vi "Calibration_Capture.vi"(8 "Detect Movement":bool, 9 "Crop?":bool, 11 "value":T1={"Pinch-valve"="Test Sample", "XLP 6000 Pump"="MRJ", "Camera1"="", "Camera2"="", "Img_Capt"=FALSE, "Actuator"=FALSE, "Pump"=FALSE, "Cam 1"=FALSE, "Cam 2"=FALSE, "Empty_Refill"=FALSE, "Crop"=FALSE, "Light intensity"=0, "Exposure Time"=0.0, "Sample Name"="", "Operator"="JFR", "Calibration 1"=path "C:/Users/au540322/Desktop/IHS_Project/images/Debris/Debris_0/Debris_0_2019_06_01-23-32-49-686.PNG", "Calibration 2"=path "C:/Users/au540322/Desktop/IHS_Project/images/Debris/Debris_0/Debris_0_2019_06_01-23-32-49-686.PNG", "Framerate"=15, "Timeout Sample"=1, "Collection date"="", "Sample size threshold"=500, "Empty start"=500, "Command"="", "Station"="", "Species Name"="", "Other Notes"="", "Aperture"=enum."Item 3", "Image Process Queue Size"=100, "Image Save Queue Size"=0, "Overload threshold"=0, "Max Framerate"=0, "Rectangle 1"={"Left"=0, "Top"=0, "Right"=0, "Bottom"=0, "Rotation"=0.0}, "Rectangle 2"={"Left"=0, "Top"=100, "Right"=100, "Bottom"=0, "Rotation"=0.0}, "Detection Region %"=200.0, "Detect 1"=path "C:/Users/au540322/Desktop/IHS_Project/images/Debris/Debris_0/Debris_0_2019_06_01-23-32-49-686.PNG", "Detect 2"=path "C:/Users/au540322/Desktop/IHS_Project/images/Debris/Debris_0/Debris_0_2019_06_01-23-32-49-686.PNG", "Max large object threshold"=500, "Open(T)/Close(F)"=FALSE, "Img_Capt Begin"=FALSE, "Dispense Speed"=0, "Flush Size"=0, "Location"="", "Latitude"="", "Longitude"="", "Determiner"="", "Sex"="", "Camera1_Img"=refnum, "Camera2_Img"=refnum, "Img1_Orig_Disp"=refnum, "Img2_Orig_Disp"=refnum, "Img1_Orig_RGB"=refnum, "Img2_Orig_RGB"=refnum, "Blue_Plane_Extract"=refnum, "Subtracted_Plane"=refnum, "Img1_Binary"=refnum, "Img2_Binary"=refnum, "Crop_Mask"=refnum, "Img1_Save"=refnum, "Img2_Save"=refnum, "Img1_Cali_Full"=refnum, "Img2_Cali_Full"=refnum, "Img1_Cali_Detect"=refnum, "Img2_Cali_Detect"=refnum, "Cam 1 queue"=refnum, "Cam 2 queue"=refnum, "Cam 1 - save queue"=refnum, "Cam 2 - save queue"=refnum, "Overlay_Ring"=0, "SystemVersion"=0, "System Serial"="", "Legacy Cam Attributes"=FALSE, "Camera Orientation 1"="", "Camera Orientation 2"="", "Pixel to mm 1"=0.0, "Pixel to mm 2"=0.0, "CAM1 Model"=enum."a2A5328-15ucBAS", "CAM2 Model"=enum."a2A5328-15ucBAS", "Flush Insect"=FALSE, "Pump Size"=TRUE, "Barcode"="", "Phase3"=FALSE, "Mega F3"="", "Container nr."=0.0, "Flush Error"=TRUE, "Start System"=FALSE, "Size Interval"=0.0, "Mun. of containers"=0.0, "Sorting sys."=FALSE, "Initial size"=0.0} {"SystemVersion" items=["Standard", "XL"]; "Overlay_Ring" items=["Session Data", "Extended Setup", "Buffer", "Camera", "Dispenser", "Stats", "Connections"]; "Flush Size" min=1; "Dispense Speed" min=1; "Rectangle 2"."Rotation" format="%.2f"; "Rectangle 2"."Left" scale=0.0..1024.0; "Rectangle 2"."Right" scale=0.0..1024.0; "Rectangle 1"."Rotation" format="%.2f"; "Rectangle 1"."Left" scale=0.0..1024.0; "Rectangle 1"."Right" scale=0.0..1024.0; "Max Framerate" min=1; "Overload threshold" min=1; "Image Save Queue Size" min=1; "Image Process Queue Size" min=1; "Empty start" min=1; "Sample size threshold" min=1; "Framerate" min=1; "Light intensity" scale=0.0..100.0}) -> (0 "Image2":T4, 1 "Image1":T4, 3 "input cluster 2":T1={"Pinch-valve"="", "XLP 6000 Pump"="", "Camera1"="", "Camera2"="", "Img_Capt"=FALSE, "Actuator"=FALSE, "Pump"=FALSE, "Cam 1"=FALSE, "Cam 2"=FALSE, "Empty_Refill"=FALSE, "Crop"=FALSE, "Light intensity"=100, "Exposure Time"=1000.0, "Sample Name"="Test Sample", "Operator"="JFR", "Calibration 1"=path "C:/Users/au540322/Desktop/IHS_Project/images/Debris/Debris_0/Debris_0_2019_06_01-23-32-49-686.PNG", "Calibration 2"=path "C:/Users/au540322/Desktop/IHS_Project/images/Debris/Debris_0/Debris_0_2019_06_01-23-32-49-686.PNG", "Framerate"=15, "Timeout Sample"=200, "Collection date"="", "Sample size threshold"=500, "Empty start"=1, "Command"="", "Station"="", "Species Name"="", "Other Notes"="", "Aperture"=enum."Item 0", "Image Process Queue Size"=500, "Image Save Queue Size"=500, "Overload threshold"=500, "Max Framerate"=100, "Rectangle 1"={"Left"=0, "Top"=0, "Right"=0, "Bottom"=0, "Rotation"=0.0}, "Rectangle 2"={"Left"=0, "Top"=0, "Right"=0, "Bottom"=0, "Rotation"=0.0}, "Detection Region %"=0.0, "Detect 1"=path "C:/Users/au540322/Desktop/IHS_Project/images/Debris/Debris_0/Debris_0_2019_06_01-23-32-49-686.PNG", "Detect 2"=path "C:/Users/au540322/Desktop/IHS_Project/images/Debris/Debris_0/Debris_0_2019_06_01-23-32-49-686.PNG", "Max large object threshold"=0, "Open(T)/Close(F)"=FALSE, "Img_Capt Begin"=FALSE, "Dispense Speed"=100, "Flush Size"=100, "Location"="Station", "Latitude"="Station", "Longitude"="Station", "Determiner"="Station", "Sex"="Station", "Camera1_Img"=refnum, "Camera2_Img"=refnum, "Img1_Orig_Disp"=refnum, "Img2_Orig_Disp"=refnum, "Img1_Orig_RGB"=refnum, "Img2_Orig_RGB"=refnum, "Blue_Plane_Extract"=refnum, "Subtracted_Plane"=refnum, "Img1_Binary"=refnum, "Img2_Binary"=refnum, "Crop_Mask"=refnum, "Img1_Save"=refnum, "Img2_Save"=refnum, "Img1_Cali_Full"=refnum, "Img2_Cali_Full"=refnum, "Img1_Cali_Detect"=refnum, "Img2_Cali_Detect"=refnum, "Cam 1 queue"=refnum, "Cam 2 queue"=refnum, "Cam 1 - save queue"=refnum, "Cam 2 - save queue"=refnum, "Overlay_Ring"=0, "SystemVersion"=0, "System Serial"="", "Legacy Cam Attributes"=FALSE, "Camera Orientation 1"="", "Camera Orientation 2"="", "Pixel to mm 1"=0.0, "Pixel to mm 2"=0.0, "CAM1 Model"=enum."a2A5328-15ucBAS", "CAM2 Model"=enum."a2A5328-15ucBAS", "Flush Insect"=FALSE, "Pump Size"=TRUE, "Barcode"="", "Phase3"=FALSE, "Mega F3"="", "Container nr."=0.0, "Flush Error"=FALSE, "Start System"=FALSE, "Size Interval"=0.0, "Mun. of containers"=0.0, "Sorting sys."=FALSE, "Initial size"=0.0} {"SystemVersion" items=["Standard", "XL"]; "Overlay_Ring" items=["Session Data", "Extended Setup", "Buffer", "Camera", "Dispenser", "Stats", "Connections"]; "Flush Size" min=1; "Dispense Speed" min=1; "Rectangle 2"."Rotation" format="%.2f"; "Rectangle 2"."Left" scale=0.0..1024.0; "Rectangle 2"."Right" scale=0.0..1024.0; "Rectangle 1"."Rotation" format="%.2f"; "Rectangle 1"."Left" scale=0.0..1024.0; "Rectangle 1"."Right" scale=0.0..1024.0; "Max Framerate" min=1; "Overload threshold" min=1; "Image Save Queue Size" min=1; "Image Process Queue Size" min=1; "Empty start" min=1; "Sample size threshold" min=1; "Framerate" min=1; "Light intensity" scale=0.0..100.0}, 4 "error out":errorcluster)   [LabVIEW 2024]
doc: "Takes calibration images with original camera aspect ratio."
uses:
  <vilib>/vision/Image Controls.llb/IMAQ Image.ctl
  controls/Data.ctl
  <vilib>/userDefined/High Color/IMAQdx.ctl
  <vilib>/vision/driver/IMAQdx.llb/IMAQdx Acquisition Mode.ctl
  <vilib>/vision/driver/NI_Vision_Acquisition_Software.lvlib
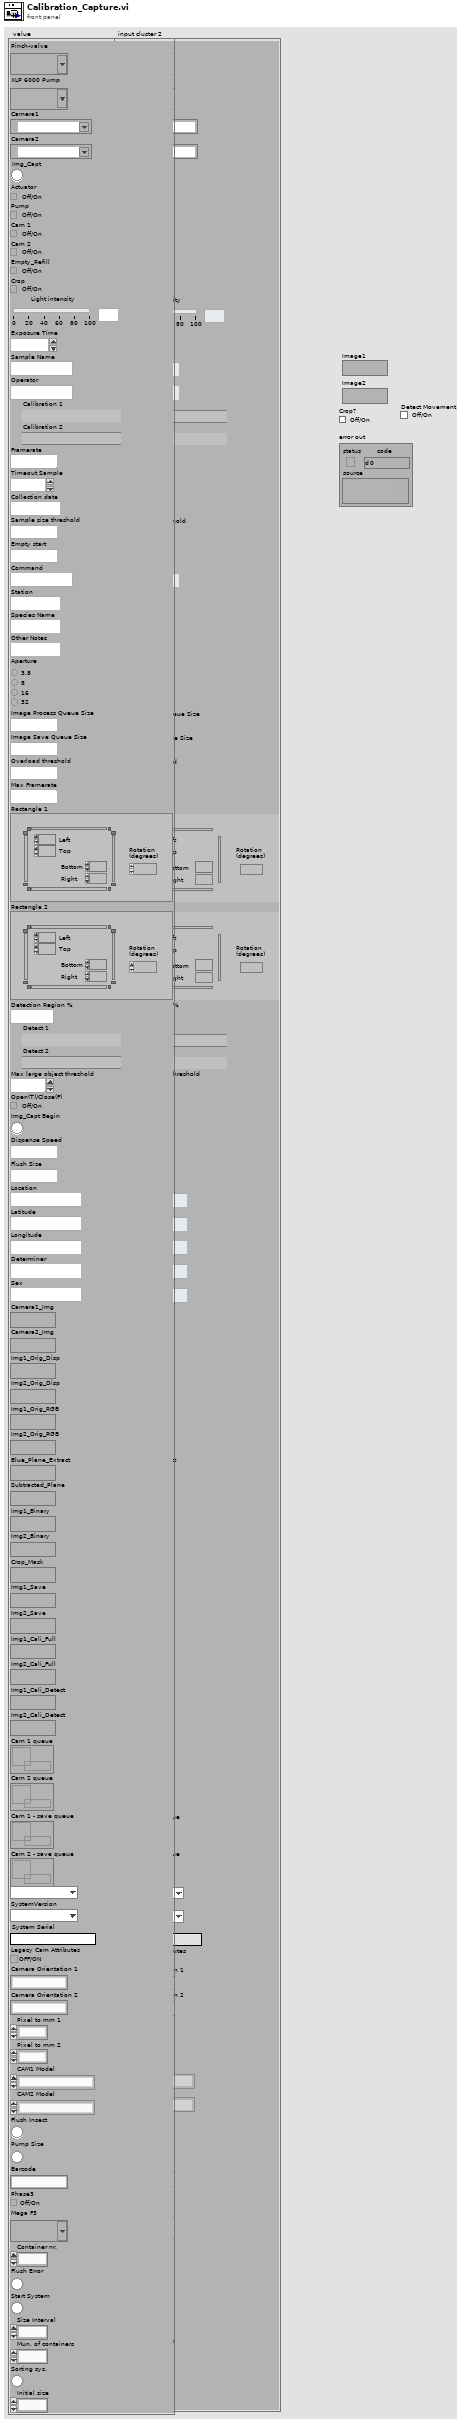
[diagram p1: front panel]
types:
  T1 = typedef "Data.ctl" = cluster{"Pinch-valve":refnum<visa-resource-name>, "XLP 6000 Pump":refnum<visa-resource-name>, "Camera1":T2, "Camera2":T2, "Img_Capt":bool, "Actuator":bool, "Pump":bool, "Cam 1":bool, "Cam 2":bool, "Empty_Refill":bool, "Crop":bool, "Light intensity":i32, "Exposure Time":dbl, "Sample Name":string, "Operator":string, "Calibration 1":path, "Calibration 2":path, "Framerate":i32, "Timeout Sample":i32, "Collection date":string, "Sample size threshold":i32, "Empty start":u32, "Command":string, "Station":string, "Species Name":string, "Other Notes":string, "Aperture":enum32{"Item 0", "Item 1", "Item 2", "Item 3"}, "Image Process Queue Size":i32, "Image Save Queue Size":i32, "Overload threshold":i32, "Max Framerate":i32, "Rectangle 1":T3, "Rectangle 2":T3, "Detection Region %":dbl, "Detect 1":path, "Detect 2":path, "Max large object threshold":i32, "Open(T)/Close(F)":bool, "Img_Capt Begin":bool, "Dispense Speed":i32, "Flush Size":i32, "Location":string, "Latitude":string, "Longitude":string, "Determiner":string, "Sex":string, "Camera1_Img":T4, "Camera2_Img":T4, "Img1_Orig_Disp":T4, "Img2_Orig_Disp":T4, "Img1_Orig_RGB":T4, "Img2_Orig_RGB":T4, "Blue_Plane_Extract":T4, "Subtracted_Plane":T4, "Img1_Binary":T4, "Img2_Binary":T4, "Crop_Mask":T4, "Img1_Save":T4, "Img2_Save":T4, "Img1_Cali_Full":T4, "Img2_Cali_Full":T4, "Img1_Cali_Detect":T4, "Img2_Cali_Detect":T4, "Cam 1 queue":refnum<queue>, "Cam 2 queue":refnum<queue>, "Cam 1 - save queue":refnum<queue>, "Cam 2 - save queue":refnum<queue>, "Overlay_Ring":u16, "SystemVersion":u16, "System Serial":string, "Legacy Cam Attributes":bool, "Camera Orientation 1":string, "Camera Orientation 2":string, "Pixel to mm 1":dbl, "Pixel to mm 2":dbl, "CAM1 Model":enum16{"a2A5328-15ucBAS", "acA1920-155uc"}, "CAM2 Model":enum16{"a2A5328-15ucBAS", "acA1920-155uc"}, "Flush Insect":bool, "Pump Size":bool, "Barcode":string, "Phase3":bool, "Mega F3":refnum<visa-resource-name>, "Container nr.":dbl, "Flush Error":bool, "Start System":bool, "Size Interval":dbl, "Mun. of containers":dbl, "Sorting sys.":bool, "Initial size":dbl}
  T2 = typedef "IMAQdx.ctl" = refnum<k21>
  T3 = typedef "IMAQ Rectangle" = cluster{"Left":i32, "Top":i32, "Right":i32, "Bottom":i32, "Rotation":dbl}
  T4 = typedef "IMAQ Image.ctl" = refnum<image>
  T5 = typedef "NI_Vision_Acquisition_Software.lvlib/IMAQdx Acquisition Mode.ctl" = enum32{"One Shot", "Continuous"}
  T6 = typedef "Image Type" = u32
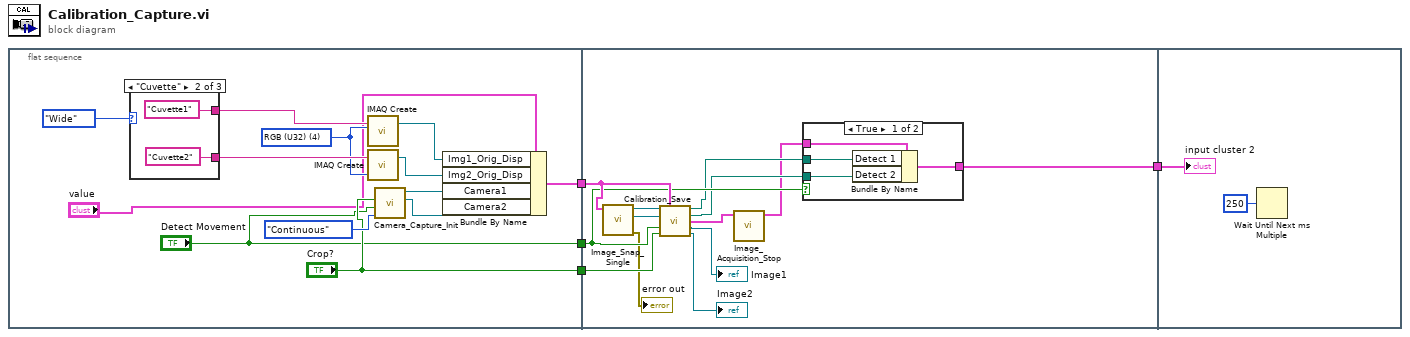
[diagram p0: block diagram]
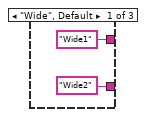
[diagram p2: hidden frame]
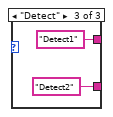
[diagram p3: hidden frame]
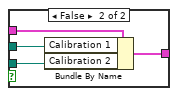
[diagram p4: hidden frame]
diagram:
  n1 = flat-sequence {
    tunnel: [w14] -> w4
    tunnel: ["Crop?"] -> w3
    tunnel: ["Detect Movement"] -> w2
    tunnel: w4 -> [w35]
    tunnel: w3 -> [w31]
    tunnel: w2 -> [w32]
    tunnel: [w36] -> w1
    tunnel: w1 -> [w46]
    frame #0 {
      w11 = T6 4 items=["Grayscale (U8)", "Grayscale (I16)", "Grayscale (SGL)", "Complex (CSG)", "RGB (U32)", "HSL (U32)", "RGB (U64)", "Grayscale (U16)"] ("Image Type")
      n2 = case shown="\"Cuvette\"" enum16{"Wide", "Cuvette", "Detect"}."Wide" {
        tunnel: ["Wide1" "Cuvette1" "Detect1"] -> w13
        tunnel: ["Wide2" "Cuvette2" "Detect2"] -> w12
        frame "Wide", Default {
        }
        frame "Cuvette" {
        }
        frame "Detect" {
        }
      }
      n3 = call "IMAQ Create"("Image Name"=w13, "Image Type"=w11) -> ("New Image"=w16:T4)  [unwired: 3 in, 1 out]
      n4 = call "IMAQ Create"("Image Name"=w12, "Image Type"=w11) -> ("New Image"=w15:T4)  [unwired: 3 in, 1 out]
      n5 = call "Camera_Capture_Init.vi"("Continuous?"=IMAQdx_Acquisition_Mode."Continuous", "Detect Movement"="Detect Movement", "Crop?"="Crop?") -> ("Camera2"=w6:T2, "Camera1"=w7:T2)  [unwired: 7 in]
      n6 = Bundle By Name(cluster="value", "Img1_Orig_Disp"=w16, "Img2_Orig_Disp"=w15, "Camera1"=w7, "Camera2"=w6) -> (w14:T1)
    }
    frame #1 {
      n7 = call "Image_Snap_Single.vi"("input cluster"=w35) -> ("error out"=→"error out":errorcluster, "Image 2"=w33:T4, "Image 1"=w34:T4)  [unwired: 7 in, 1 out]
      n8 = call "Calibration_Save.vi"("Img1"=w34, "Data"=w35, "Img2"=w33, "Dtct"=w32, "Crop?"=w31) -> ("Cal1"=w29:path, "Cal2"=w28:path, "Data out"=w24:T1, "Img1 out"=→"Image1":T4, "Img2 out"=→"Image2":T4)  [unwired: 6 in]
      n9 = call "Image_Acquisition_Stop.vi"("input cluster"=w24) -> ("input cluster 2"=w25:T1)  [unwired: 9 in, 1 out]
      n10 = case shown="True" w32 {
        tunnel: w25 -> [w40 w44]
        tunnel: [w39 w43] -> w36
        tunnel: w28 -> [w38 w42]
        tunnel: w29 -> [w37 w41]
        frame True {
          n11 = Bundle By Name(cluster=w40, "Detect 1"=w37, "Detect 2"=w38) -> (w39:T1)
        }
        frame False {
          n12 = Bundle By Name(cluster=w44, "Calibration 1"=w41, "Calibration 2"=w42) -> (w43:T1)
        }
      }
    }
    frame #2 {
      n13 = Wait Until Next ms Multiple(millisecond multiple=u32 250) -> ()  [unwired: 1 out]
      "input cluster 2" <- w46
    }
  }
